vi "get_overlay.vi"(4 "error in (no error)":errorcluster, 6 "Container State":T9, 7 "Display State In":T1 {"array of overlays"."overlay size" min=1}) -> (0 "error out":errorcluster, 2 "Value":T6={"overlay array"=[], "overlay name"="", "color (red)"=16711680, "overlay size"=0, "overlay type"=enum."crosshair"} {"overlay size" min=1}, 3 "Display State Out":T1 {"array of overlays"."overlay size" min=1})   [LabVIEW 2010, in "XImage.xctl"]
uses:
  XImage.xctl
  <vilib>/_xctls/Container State.ctl
  <vilib>/_xctls/XControlSupport.lvlib
  ROI_frames_cluster.ctl
  enumerations/unit.ctl
  classes/Image/Image/Image.lvclass
  calibration_cluster.ctl
  xpath_cluster.ctl
  classes/SpaceVector/SpaceVector/SpaceVector.lvclass
  overlays_cluster.ctl
  classes/PointCollection/PointCollection/PointCollection.lvclass
  ROI_mode_enum.ctl
  last_action_enum.ctl
  state.ctl
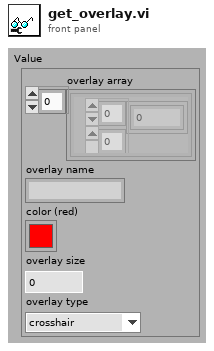
[diagram p1: front panel]
types:
  T1 = typedef "XImage.xctl/state.ctl" = cluster{"current frame index":i32, "number of images":i32, "ROI (frames)":T2, "control refs":cluster{"frame":refnum<vi>, "image":refnum<vi>, "saveROIsButton":refnum<vi>, "loadImageSwitch":refnum<vi>, "loadROIsSwitch":refnum<vi>, "saveROIsSwitch":refnum<vi>, "loadImagePath":refnum<vi>, "loadROIPath":refnum<vi>}, "calibration":T3, "xpaths":T5, "offset":refnum<class "SpaceVector.lvclass">, "XML description":string, "number of ROIs":dbl, "ROI Tool Buttons Visible":cluster{"Zoom Tool":bool, "Selection Tool":bool, "Pan Tool":bool, "Point Tool":bool, "Line Tool":bool, "Rectangle Tool":bool, "Rotated Rectangle Tool":bool, "Polyline Tool":bool, "Polygon Tool":bool, "Freehand Tool":bool, "Closed Freehand Tool":bool, "Ellipse Tool":bool, "Annulus Tool":bool}, "ROI color":u32, "number color":u32, "enable ROI numbering?":bool, "selected path to save ROIs":path, "starting path":path, "array of overlays":T6[], "pointCollection":refnum<class "PointCollection.lvclass">, "ROImode":T7, "selected point ID":dbl, "point radius":i32, "point colours":u32[], "ROI info":variant, "PlotAreaSize":cluster{"Width":u32, "Height":u32}, "last action":T8}
  T2 = typedef "XImage.xctl/ROI_frames_cluster.ctl" = cluster{"ROI":cluster{"Global Rectangle":i32[], "Contours":cluster{"Contour Type":u32, "ROI Type":u32, "Points":i32[]}[]}[]}
  T3 = typedef "XImage.xctl/calibration_cluster.ctl" = cluster{"x":dbl, "y":dbl, "x unit":T4, "y unit":T4}
  T4 = typedef "Image.lvclass/unit.ctl" = enum16{"um", "s"}
  T5 = typedef "XImage.xctl/xpath_cluster.ctl" = cluster{"x offset":string, "y offset":string, "z offset":string}
  T6 = typedef "XImage.xctl/overlays_cluster.ctl" = cluster{"overlay array":cluster{i32[][]}[], "overlay name":string, "color (red)":u32, "overlay size":i32, "overlay type":enum16{"crosshair", "circle"}}
  T7 = typedef "XImage.xctl/ROI_mode_enum.ctl" = enum16{"none", "IMAQROIs", "PointCollection"}
  T8 = typedef "XImage.xctl/last_action_enum.ctl" = enum16{"not specified", "image loaded", "frame changed", "ROIs changed"}
  T9 = typedef "XControlSupport.lvlib/Container State.ctl" = cluster{"Indicator?":bool, "Run Mode?":bool, " Refnum":refnum<vi>}
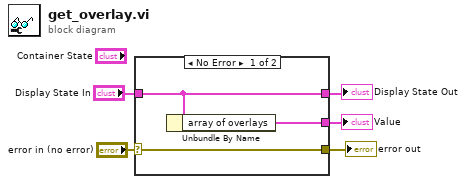
[diagram p0: block diagram]
diagram:
  n1 = case shown="No Error" "error in (no error)" {
    selector: "error in (no error)" -> [w7 w10]
    tunnel: [w7 w10] -> w1
    tunnel: "Display State In" -> [w8 w9]
    tunnel: [w8 w9] -> w2
    tunnel: [w6 _] -> w3
    frame No Error {
      n2 = Unbundle By Name(w8) -> ("array of overlays"=w6:T6[])
    }
    frame Error {
    }
  }
  "error out" <- w1
  "Value" <- w3
  "Display State Out" <- w2
